vi "Merge Cluster.vi"(8 "error in (no error)":errorcluster, 10 "Claster to Merge":T1, 11 "Main Cluster":T1) -> (0 "error out":errorcluster, 3 "Merged Main Cluster":T1)   [LabVIEW 2019, in "Core.lvlib" / "Core.lvclass"]
uses:
  Core.lvclass
  <vilib>/ActorFramework/Message Enqueuer/Message Enqueuer.lvclass
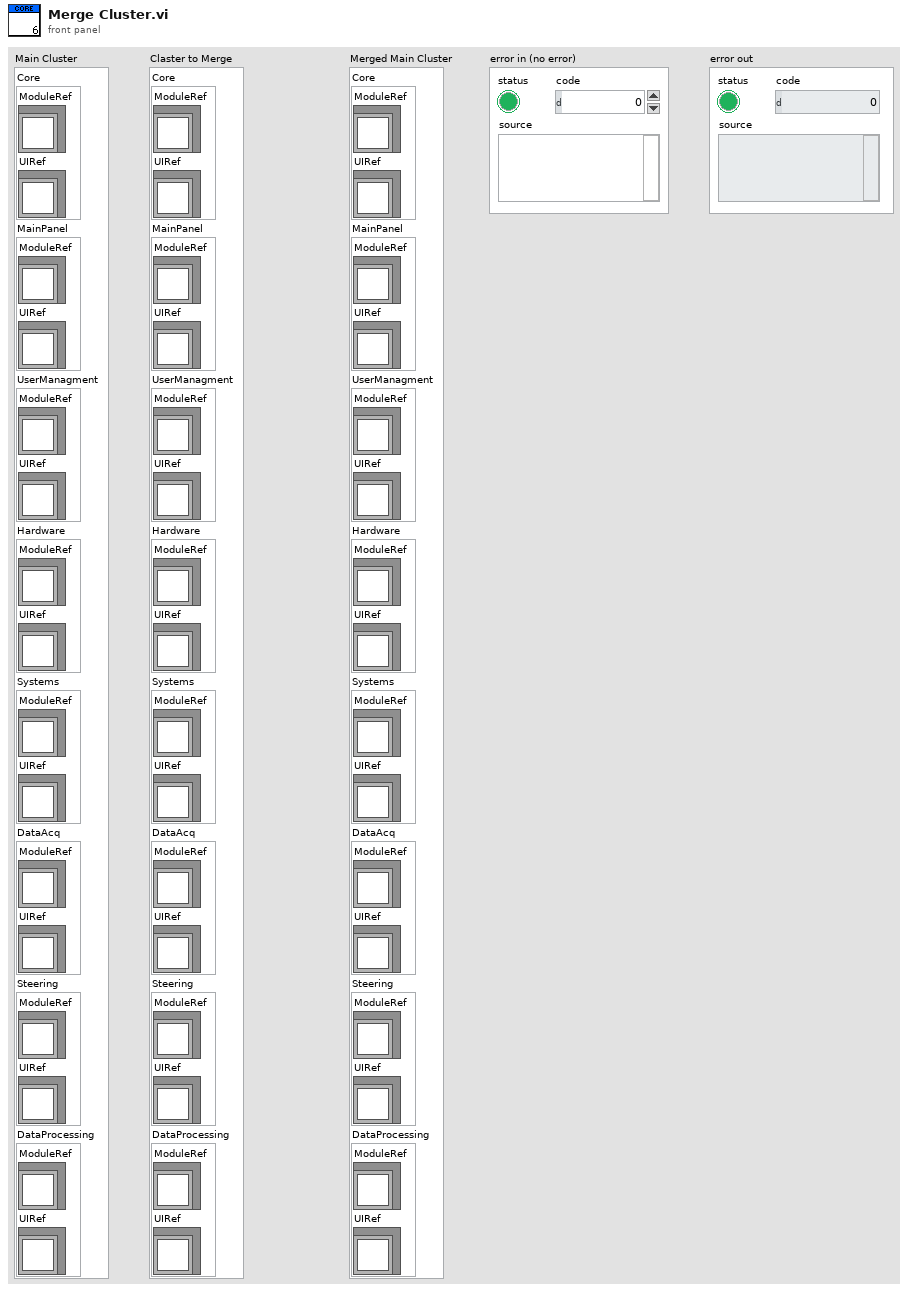
[diagram p1: front panel]
types:
  T1 = cluster{"Core":cluster{"ModuleRef":refnum<class "Message Enqueuer.lvclass">, "UIRef":refnum<class "Message Enqueuer.lvclass">}, "MainPanel":cluster{"ModuleRef":refnum<class "Message Enqueuer.lvclass">, "UIRef":refnum<class "Message Enqueuer.lvclass">}, "UserManagment":cluster{"ModuleRef":refnum<class "Message Enqueuer.lvclass">, "UIRef":refnum<class "Message Enqueuer.lvclass">}, "Hardware":cluster{"ModuleRef":refnum<class "Message Enqueuer.lvclass">, "UIRef":refnum<class "Message Enqueuer.lvclass">}, "Systems":cluster{"ModuleRef":refnum<class "Message Enqueuer.lvclass">, "UIRef":refnum<class "Message Enqueuer.lvclass">}, "DataAcq":cluster{"ModuleRef":refnum<class "Message Enqueuer.lvclass">, "UIRef":refnum<class "Message Enqueuer.lvclass">}, "Steering":cluster{"ModuleRef":refnum<class "Message Enqueuer.lvclass">, "UIRef":refnum<class "Message Enqueuer.lvclass">}, "DataProcessing":cluster{"ModuleRef":refnum<class "Message Enqueuer.lvclass">, "UIRef":refnum<class "Message Enqueuer.lvclass">}}
  T2 = cluster{"ModuleRef":refnum<class "Message Enqueuer.lvclass">, "UIRef":refnum<class "Message Enqueuer.lvclass">}[]
  T3 = cluster{"ModuleRef":refnum<class "Message Enqueuer.lvclass">, "UIRef":refnum<class "Message Enqueuer.lvclass">}
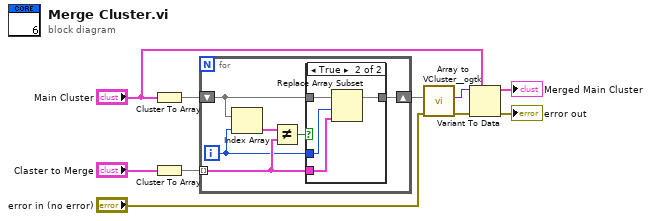
[diagram p0: block diagram]
diagram:
  n1 = Cluster To Array(cluster="Main Cluster") -> (array=w3:T2)
  n2 = Cluster To Array(cluster="Claster to Merge") -> (array=w2:T2)
  n3 = for {
    tunnel: w2 -> [w15] mode=indexing
    shift-right: [w12] -> w4
    shift-left: w3 -> [w13]
    i -> [w11]
    n4 = Index Array(array=w13, index=w11) -> (element=w14:T3)
    n5 = Not Equal?(x=w14, y=w15) -> (x != y?=w16:bool)
    n6 = case shown="True" w16 {
      tunnel: w15 -> [_ w18]
      tunnel: w13 -> [w17 w21]
      tunnel: [w17 w20] -> w12
      tunnel: w11 -> [_ w19]
      frame False {
      }
      frame True {
        n7 = Replace Array Subset(array=w21, new element=w18, index=w19) -> (w20:T2)
      }
    }
  }
  n8 = call <userlib>:"Array to VCluster__ogtk.vi"("error in (no error)"="error in (no error)", "Array"=w4) -> ("error out"=w5:errorcluster, "VCluster"=w6:variant)  [unwired: 8 in]
  n9 = Variant To Data(error in=w5, type="Main Cluster", Variant=w6) -> (data=→"Merged Main Cluster":T1, error out=→"error out":errorcluster)
